vi "UI_AutoRefresh_Init.vi"(8 "error in (no error)":errorcluster, 10 "Parameters":T1={"Write TipStrips with details (T)"=TRUE, "Write Captions with UserLabels (T)"=TRUE, "Mode (ind only)"=enum."Indicators only", "Enable nested stream (T)"=TRUE}, 11 "UIA_UTsupport in":refnum<class "UIA_UTsupport.lvclass">) -> (0 "error out":errorcluster, 3 "UIA_UTsupport out":refnum<class "UIA_UTsupport.lvclass">)   [LabVIEW 2020, in "UIA_UTsupport.lvlib" / "UIA_UTsupport.lvclass"]
uses:
  UIA_UTsupport.lvclass
  UI_Actor/UI_Actor/ctl_AR_Parameters.ctl
  UI_Actor/UI_Actor/ctl_AR_Mode.ctl
  gloglo.vi
  UI_Actor/UI_Actor/UI_Actor.lvclass
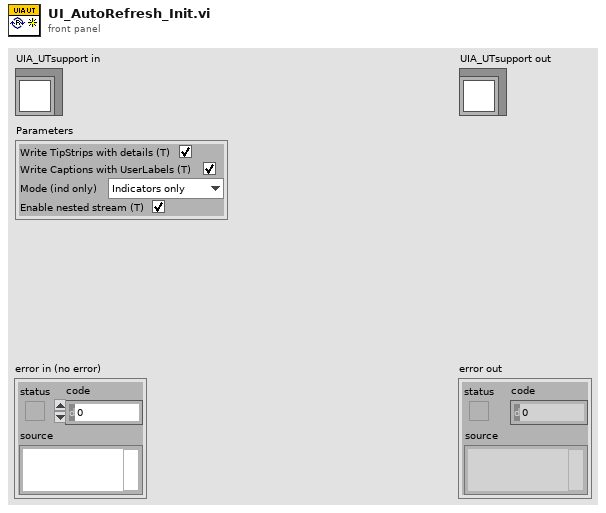
[diagram p1: front panel]
types:
  T1 = typedef "UI_Actor.lvlib/UI_Actor.lvclass/ctl_AR_Parameters.ctl" = cluster{"Write TipStrips with details (T)":bool, "Write Captions with UserLabels (T)":bool, "Mode (ind only)":T2, "Enable nested stream (T)":bool}
  T2 = typedef "UI_Actor.lvlib/UI_Actor.lvclass/ctl_AR_Mode.ctl" = enum16{"Controls only", "Indicators only", "All"}
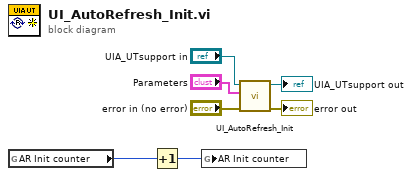
[diagram p0: block diagram]
diagram:
  n1 = global read "gloglo.vi" "AR Init counter"() -> (w2:i32)
  n2 = Increment(x=w2) -> (x+1=w1:i32)
  n3 = global write "gloglo.vi" "AR Init counter"(w1) -> ()
  n4 = call-parent "UI_AutoRefresh_Init.vi"("error in (no error)"="error in (no error)", "Parameters"="Parameters", "UI_Actor in"="UIA_UTsupport in") -> ("error out"=→"error out":errorcluster, "UI_Actor out"=→"UIA_UTsupport out":refnum<class "UIA_UTsupport.lvclass">)  [unwired: 7 in]
